vi "Static Preallocated.vi"(8 "error in (no error)":errorcluster, 11 "Test Class in":refnum<class "Test Class.lvclass">) -> (0 "error out":errorcluster, 2 "dt out (s)":dbl, 3 "Test Class out":refnum<class "Test Class.lvclass">)   [LabVIEW 2024, in "Test Class.lvclass"]
uses:
  Test Class.lvclass
  Test Class.lvclass/Test Class.ctl
  <vilib>/addons/control/pid/NI_PID_pid.lvlib
  <vilib>/addons/control/pid/pid.llb/PID (DBL).vi
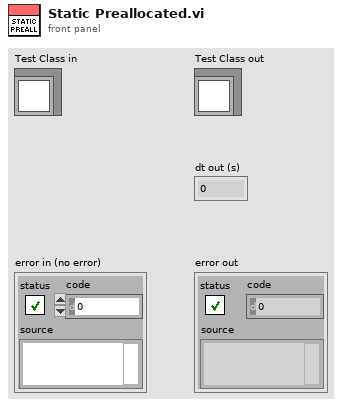
[diagram p1: front panel]
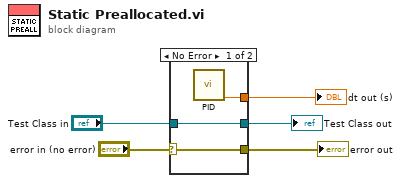
[diagram p0: block diagram]
diagram:
  n1 = case shown="No Error" "error in (no error)" {
    selector: "error in (no error)" -> [w7 w10]
    tunnel: [w7 w10] -> w4
    tunnel: [w8 w9] -> w2
    tunnel: "Test Class in" -> [w8 w9]
    tunnel: [w6 _] -> w1
    frame No Error {
      n2 = call-poly <vilib>:"PID.vi"() -> ("dt out (s)"=w6:dbl)  [unwired: 10 in, 1 out]
    }
    frame Error {
    }
  }
  "error out" <- w4
  "Test Class out" <- w2
  "dt out (s)" <- w1
